vi "OE1022D_Configure Reference Source.vi"(0 "VISA resource name":refnum<visa-resource-name>, 1 "OE1022D A/B":u8(ring) items=["Channel A", "Channel B"], 2 "Reference Source":u8(ring) items=["External", "Internal", "Internal Sweep"], 5 "error in (no error)":errorcluster) -> (14 "VISA resource name out":refnum<visa-resource-name>, 19 "error out":errorcluster)   [LabVIEW 2024]
doc: "Configures the reference source and the internal oscillator."
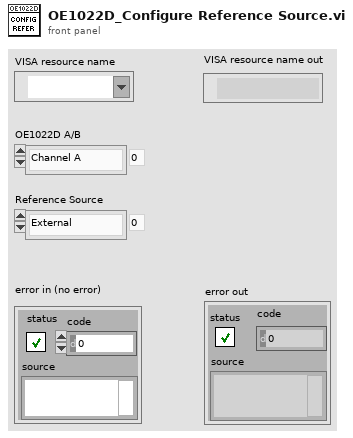
[diagram p1: front panel]
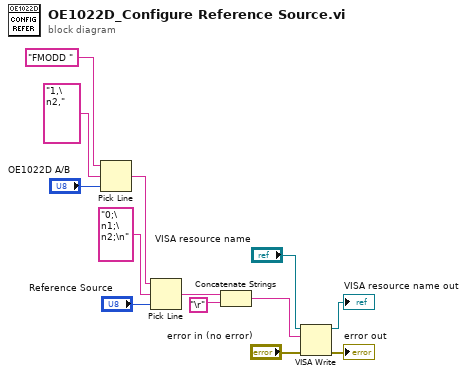
[diagram p0: block diagram]
diagram:
  n1 = Pick Line(string ("")="FMODD ", multi-line string="1,\n2,", line index="OE1022D A/B") -> (output string=w13:string)
  n2 = Pick Line(string ("")=w13, multi-line string="0;\n1;\n2;\n", line index="Reference Source") -> (output string=w2:string)
  n3 = Concatenate Strings(w2, "\r") -> (w1:string)
  n4 = VISA Write(VISA resource name="VISA resource name", write buffer=w1, error in (no error)="error in (no error)") -> (VISA resource name out=→"VISA resource name out":refnum<visa-resource-name>, error out=→"error out":errorcluster)  [unwired: 1 out]
